vi "setScanState.vi"(8 "error in (no error)":errorcluster, 10 "Scan State":T1, 11 "Inst.Xeryon-Rotator in":refnum<class "Inst.Xeryon-Rotator.lvclass">) -> (0 "error out":errorcluster, 3 "Inst.Xeryon-Rotator out":refnum<class "Inst.Xeryon-Rotator.lvclass">)   [LabVIEW 2019, in "Inst.Xeryon-Rotator.lvclass"]
doc: "Scan Left = Decrease Angle\nScan Right = Increase Angle"
uses:
  Inst.Xeryon-Rotator.lvclass
  Typedefs/Inst.Xeryon-Rotator.Commands--Enum.ctl
  <userlib>/LevyLab/Instrument Framework/Instrument/Instrument.lvclass
  C:/Program Files (x86)/National Instruments/LabVIEW 2019/user.lib/LevyLab/Instrument Framework/Instrument/Instrument.lvclass
  Typedefs/Inst.Xeryon-Rotator.ScanState--Enum.ctl
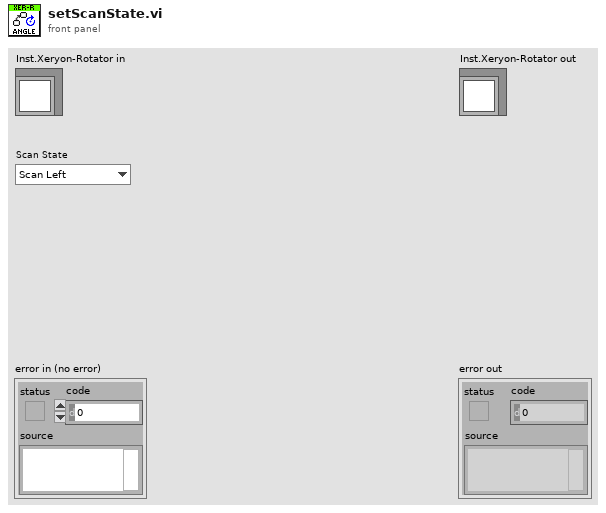
[diagram p1: front panel]
types:
  T1 = typedef "Inst.Xeryon-Rotator.lvclass/Inst.Xeryon-Rotator.ScanState--Enum.ctl" = enum16{"Scan Left", "Stop", "Scan Right"}
  T2 = typedef "Inst.Xeryon-Rotator.lvclass/Inst.Xeryon-Rotator.Commands--Enum.ctl" = enum16{"setAngle", "getAngle", "setState"}
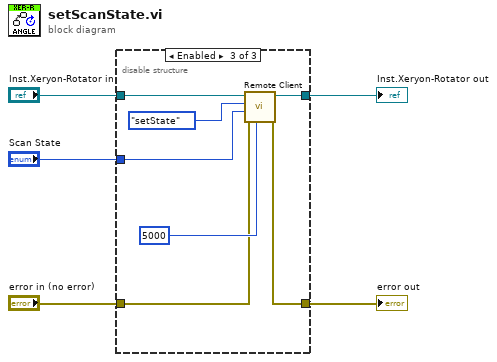
[diagram p0: block diagram]
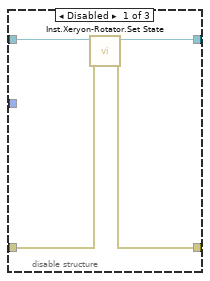
[diagram p2: hidden frame]
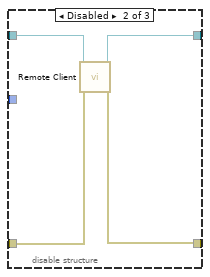
[diagram p3: hidden frame]
diagram:
  n1 = disable-structure shown="Enabled" {
    disable-tunnel: "Inst.Xeryon-Rotator in" -> [w9 w13 w19]
    disable-tunnel: "error in (no error)" -> [w8 w11 w16]
    disable-tunnel: [w7 w10 w17] -> w3
    disable-tunnel: [w6 w12 w18] -> w2
    disable-tunnel: "Scan State" -> [_ _ w14]
    frame Disabled {
      n2 = call "Inst.Xeryon-Rotator.Set State.vi"("error in (no error)"=w8, "Inst.Xeryon-Rotator in"=w9) -> ("error out"=w7:errorcluster, "Inst.Xeryon-Rotator out"=w6:refnum<class "Inst.Xeryon-Rotator.lvclass">)  [unwired: 8 in]
    }
    frame Disabled {
      n3 = call <userlib>:"Remote Client.vi"("error in (no error)"=w11, "Instrument in"=w13) -> ("error out"=w10:errorcluster, "Instrument out"=w12:refnum<class "Inst.Xeryon-Rotator.lvclass">)  [unwired: 6 in, 2 out]
    }
    frame Enabled {
      n4 = call <userlib>:"Remote Client.vi"("timeout (ms) [500]"=5000, "error in (no error)"=w16, "Data in"=w14, "Command in"=Inst.Xeryon-Rotator.Commands--Enum."setState" ("Commands"), "Instrument in"=w19) -> ("error out"=w17:errorcluster, "Instrument out"=w18:refnum<class "Inst.Xeryon-Rotator.lvclass">)  [unwired: 3 in, 2 out]
    }
  }
  "error out" <- w3
  "Inst.Xeryon-Rotator out" <- w2
